vi "Run.vi"(8 "error in (no error)":errorcluster, 9 "Penalty":dbl, 10 "Maze (0: Empty, -1: Enemy. 1: Teammate":i32[][](array[numeric]), 11 "Runner in":refnum<class "Shield Wall.lvclass">) -> (0 "error out":errorcluster, 1 "Direction":T1, 2 "Action":T2, 3 "Runner out":refnum<class "Shield Wall.lvclass">, 4 "Replicated":refnum<class "Square.lvclass">)   [LabVIEW 2015, in "Shield Wall.lvclass"]
uses:
  Shield Wall.lvclass
  Type Defs/Action Enum.ctl
  Type Defs/Direction Enum.ctl
  Square/Square.lvclass
  DVR Cluster.ctl
  Shield Wall.lvclass/Shield Wall.ctl
  SubVIs/Read-Only Globals.vi
  Type Defs/SB Type Defs.lvlib
panel:
  # "NOTICE - YOU MUST NOT REMOVE THIS NOTICE. PER THE FOLLOWING LICENSE, YOU MAY REPRODUCE THIS SOFTWARE PROVIDED YOU FOLLOW THE TERMS\nOF THE LICENSE.\n\n---BEGIN BSD LICENSE (http://opensource.org/licenses/BSD-2-Clause)---\nCopyright (c) 2015, Endigit, Inc. <robert@endigit.com>\nAll rights reserved.\n\nRedistribution and use in source and binary forms, with or without modification, are permitted provided that the following conditions are met:\n\n1. Redistributions of source code must retain the above copyright notice, this list of conditions and the following disclaimer.\n\n2. Redistributions in binary form must reproduce the above copyright notice, this list of conditions and the following disclaimer in the documentation and/or other \nmaterials provided with the distribution.\n\nTHIS SOFTWARE IS PROVIDED BY THE COPYRIGHT HOLDERS AND CONTRIBUTORS \"AS IS\" AND ANY EXPRESS OR IMPLIED WARRANTIES, INCLUDING, BUT NOT \nLIMITED TO, THE IMPLIED WARRANTIES OF MERCHANTABILITY AND FITNESS FOR A PARTICULAR PURPOSE ARE DISCLAIMED. IN NO EVENT SHALL THE COPYRIGHT \nHOLDER OR CONTRIBUTORS BE LIABLE FOR ANY DIRECT, INDIRECT, INCIDENTAL, SPECIAL, EXEMPLARY, OR CONSEQUENTIAL DAMAGES (INCLUDING, BUT NOT \nLIMITED TO, PROCUREMENT OF SUBSTITUTE GOODS OR SERVICES; LOSS OF USE, DATA, OR PROFITS; OR BUSINESS INTERRUPTION) HOWEVER CAUSED AND ON \nANY THEORY OF LIABILITY, WHETHER IN CONTRACT, STRICT LIABILITY, OR TORT (INCLUDING NEGLIGENCE OR OTHERWISE) ARISING IN ANY WAY OUT OF THE USE \nOF THIS SOFTWARE, EVEN IF ADVISED OF THE POSSIBILITY OF SUCH DAMAGE.\n---END BSD LICENSE---"
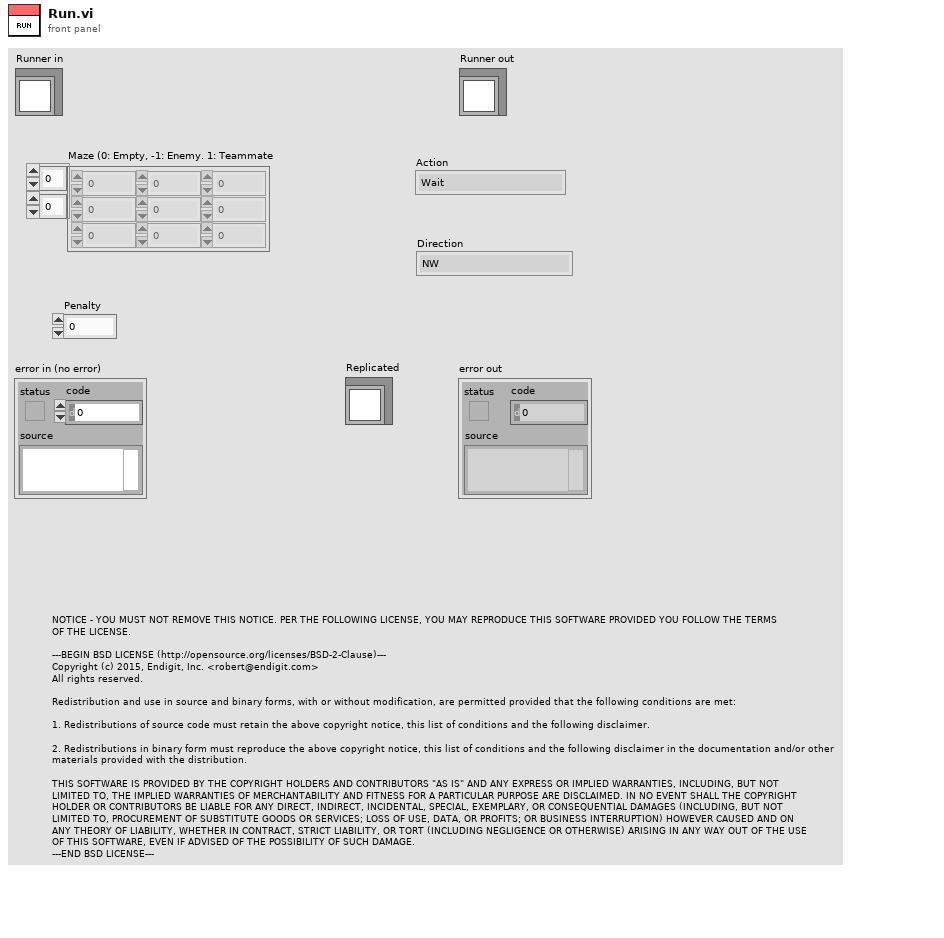
[diagram p1: front panel]
types:
  T1 = typedef "SB Type Defs.lvlib/Direction Enum.ctl" = enum16{"NW", "N", "NE", "E", "SE", "S", "SW", "W"}
  T2 = typedef "SB Type Defs.lvlib/Action Enum.ctl" = enum16{"Wait", "Move", "Attack", "Replicate"}
  T3 = typedef "Shield Wall.lvclass/DVR Cluster.ctl" = cluster{"N":i32, "E":i32, "S":i32, "W":i32, "Init":bool, "R":i32}
  T4 = typedef "Shield Wall.lvclass/Post Enum.ctl" = enum16{"NW", "NNW", "NNE", "NE", "ENE", "ESE", "SE", "SSE", "SSW", "SW", "WSW", "WNW"}
  T5 = typedef "Shield Wall.lvclass/Ring Enum.ctl" = enum16{"Defense", "Fill", "Hold", "Spawn", "Replicate", "Inner"}
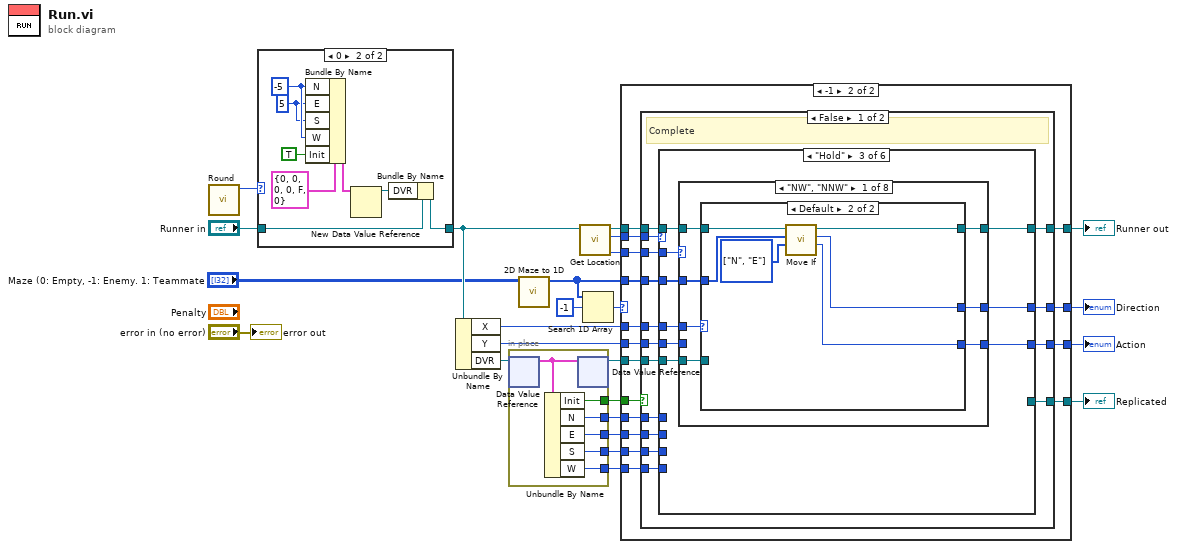
[diagram p0: block diagram]
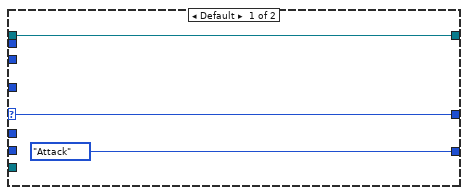
[diagram p2: hidden frame]
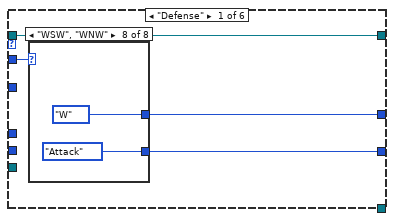
[diagram p3: hidden frame]
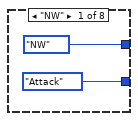
[diagram p4: hidden frame]
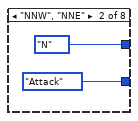
[diagram p5: hidden frame]
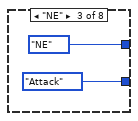
[diagram p6: hidden frame]
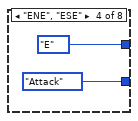
[diagram p7: hidden frame]
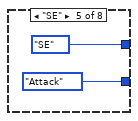
[diagram p8: hidden frame]
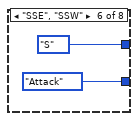
[diagram p9: hidden frame]
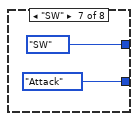
[diagram p10: hidden frame]
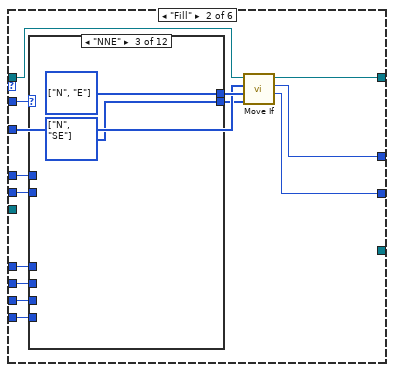
[diagram p11: hidden frame]
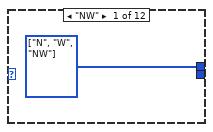
[diagram p12: hidden frame]
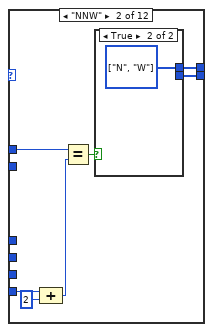
[diagram p13: hidden frame]
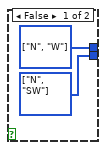
[diagram p14: hidden frame]
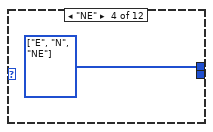
[diagram p15: hidden frame]
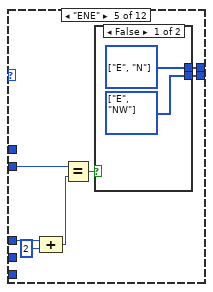
[diagram p16: hidden frame]
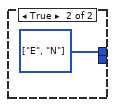
[diagram p17: hidden frame]
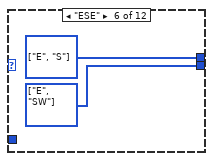
[diagram p18: hidden frame]
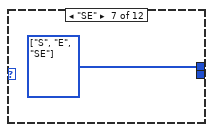
[diagram p19: hidden frame]
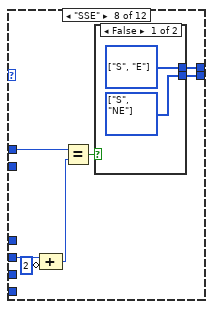
[diagram p20: hidden frame]
diagram:
  n1 = call "Round.vi"() -> ("Round"=w23:i32)  [unwired: 11 in]
  n2 = case shown="0" w23 {
    tunnel: "Runner in" -> [w25 w33]
    tunnel: [w25 w31] -> w20
    frame Default {
    }
    frame 0 {
      w27 = 5 ("E")
      w28 = -5 ("N")
      n3 = Bundle By Name(cluster=T3 {"N"=0, "E"=0, "S"=0, "W"=0, "Init"=FALSE, "R"=0} ("DVR Cluster"), "N"=w28, "E"=w27, "S"=w27, "W"=w28, "Init"=TRUE) -> (w29:T3)
      n4 = New Data Value Reference(data value=w29) -> (data value reference=w32:refnum<data-value>)  [unwired: 1 in, 1 out]
      n5 = Bundle By Name(cluster=w33, "DVR"=w32) -> (w31:refnum<class "Shield Wall.lvclass">)
    }
  }
  n6 = Unbundle By Name(w20) -> ("X"=w18:i32, "Y"=w17:i32, "DVR"=w21:refnum<data-value>)
  n7 = in-place {
    in-place-border: [w38] -> w16
    in-place-border: [w37] -> w7
    in-place-border: [w36] -> w6
    in-place-border: [w35] -> w5
    in-place-border: [w34] -> w4
    n8 = in-place-dvr #1(w21) -> (w39:T3)  [unwired: 1 out]
    n9 = Unbundle By Name(w39) -> ("Init"=w38:bool, "N"=w37:i32, "E"=w36:i32, "S"=w35:i32, "W"=w34:i32)
    n10 = in-place-dvr #1(w39) -> (w11:refnum<data-value>)  [unwired: 1 out]
  }
  n11 = call "2D Maze to 1D.vi"("Maze (0: Empty, -1: Enemy. >0: Teammate"="Maze (0: Empty, -1: Enemy. 1: Teammate") -> ("1D Maze"=w9:i32[])  [unwired: 10 in]
  n12 = call "Get Location.vi"("Class"=w20) -> ("Post"=w1:T4, "Ring"=w2:T5, "Class"=w3:refnum<class "Shield Wall.lvclass">)  [unwired: 8 in]
  n13 = Search 1D Array(1D array=w9, element=-1) -> (index of element=w8:i32)  [unwired: 1 in]
  n14 = case shown="-1" w8 {
    selector: w8 -> [w40 _]
    tunnel: w3 -> [w42 w58]
    tunnel: [w42 w57] -> w19
    tunnel: w18 -> [_ w56]
    tunnel: w17 -> [_ w55]
    tunnel: w16 -> [_ w54]
    tunnel: [w40 w53] -> w15
    tunnel: [Action_Enum."Attack" ("Action") w52] -> w14
    tunnel: [_ w51] -> w13
    tunnel: w11 -> [_ w50]
    tunnel: w9 -> [_ w49]
    tunnel: w7 -> [_ w48]
    tunnel: w6 -> [_ w47]
    tunnel: w5 -> [_ w46]
    tunnel: w4 -> [_ w45]
    tunnel: w2 -> [_ w44]
    tunnel: w1 -> [_ w43]
    frame Default {
    }
    frame -1 {
      n15 = case shown="False" w54 {
        tunnel: w58 -> [w72 w448]
        tunnel: [w73 w444] -> w57
        tunnel: w56 -> [w60 w450]
        tunnel: w55 -> [w59 w451]
        tunnel: w49 -> [w69 w449]
        tunnel: [w68 w445] -> w53
        tunnel: [w67 w446] -> w52
        tunnel: w50 -> [w65 w447]
        tunnel: [w66 w443] -> w51
        tunnel: w48 -> [w64 _]
        tunnel: w47 -> [w63 _]
        tunnel: w46 -> [w62 _]
        tunnel: w45 -> [w61 _]
        tunnel: w44 -> [w71 _]
        tunnel: w43 -> [w70 _]
        frame False {
          # "Complete"
          n16 = case shown="\"Hold\"" w71 {
            tunnel: [w77 w100 w163 w324 w343 w418] -> w73
            tunnel: w72 -> [w77 w96 w166 w320 w346 w416]
            tunnel: w70 -> [w74 w107 w168 w319 w341 _]
            tunnel: w69 -> [_ w95 w167 w321 w347 w421]
            tunnel: [w75 w99 w164 w322 w344 w420] -> w68
            tunnel: [w76 w98 w165 w323 w345 w419] -> w67
            tunnel: [_ _ _ _ w342 _] -> w66
            tunnel: w65 -> [_ _ w160 _ _ _]
            tunnel: w64 -> [_ w103 _ _ _ _]
            tunnel: w63 -> [_ w102 _ _ _ _]
            tunnel: w62 -> [_ w101 _ _ _ _]
            tunnel: w61 -> [_ w104 _ _ _ _]
            tunnel: w60 -> [_ w106 w162 _ _ _]
            tunnel: w59 -> [_ w105 w161 _ _ _]
            frame "Defense" {
              n17 = case shown="\"WSW\", \"WNW\"" w74 {
                tunnel: [Action_Enum."Attack" ("Action") Action_Enum."Attack" ("Action") Action_Enum."Attack" ("Action") Action_Enum."Attack" ("Action") Action_Enum."Attack" ("Action") Action_Enum."Attack" ("Action") Action_Enum."Attack" ("Action") Action_Enum."Attack" ("Action")] -> w76
                tunnel: [Direction_Enum."NW" ("Direction") Direction_Enum."N" ("Direction") Direction_Enum."NE" ("Direction") Direction_Enum."E" ("Direction") Direction_Enum."SE" ("Direction") Direction_Enum."S" ("Direction") Direction_Enum."SW" ("Direction") Direction_Enum."W" ("Direction")] -> w75
                frame "NW" {
                }
                frame "NNW", "NNE" {
                }
                frame "NE" {
                }
                frame "ENE", "ESE" {
                }
                frame "SE" {
                }
                frame "SSE", "SSW" {
                }
                frame "SW" {
                }
                frame "WSW", "WNW" {
                }
              }
            }
            frame "Fill" {
              n18 = case shown="\"NNE\"" w107 {
                tunnel: w106 -> [_ w113 _ _ _ _ _ w140 _ _ _ _]
                tunnel: w105 -> [_ _ _ _ w124 _ _ _ _ _ w151 _]
                tunnel: w104 -> [_ w115 _ _ _ _ _ _ _ _ _ _]
                tunnel: w103 -> [_ _ _ _ w125 _ _ _ _ _ _ _]
                tunnel: w102 -> [_ _ _ _ _ _ _ w137 _ _ _ _]
                tunnel: w101 -> [_ _ _ _ _ _ _ _ _ _ w150 _]
                tunnel: [w108 w110 w120 w121 w123 w133 w134 w136 w146 w147 w149 w159] -> w97
                tunnel: [_ w109 w119 _ w122 w132 _ w135 w145 _ w148 w158] -> w94
                frame "NW" {
                  w108 = T1[] [enum."N", enum."W", enum."NW"] items=["NW", "N", "NE", "E", "SE", "S", "SW", "W"]
                }
                frame "NNW" {
                  n19 = Compound Arithmetic op=ADD(w115, 2 ("value")) -> (w111:i32)
                  n20 = Equal?(x=w113, y=w111) -> (x = y?=w112:bool)
                  n21 = case shown="True" w112 {
                    tunnel: [w117 w118] -> w110
                    tunnel: [w116 _] -> w109
                    frame False {
                      w116 = T1[] [enum."N", enum."SW"] items=["NW", "N", "NE", "E", "SE", "S", "SW", "W"]
                      w117 = T1[] [enum."N", enum."W"] items=["NW", "N", "NE", "E", "SE", "S", "SW", "W"]
                    }
                    frame True {
                      w118 = T1[] [enum."N", enum."W"] items=["NW", "N", "NE", "E", "SE", "S", "SW", "W"]
                    }
                  }
                }
                frame "NNE" {
                  w119 = T1[] [enum."N", enum."SE"] items=["NW", "N", "NE", "E", "SE", "S", "SW", "W"]
                  w120 = T1[] [enum."N", enum."E"] items=["NW", "N", "NE", "E", "SE", "S", "SW", "W"]
                }
                frame "NE" {
                  w121 = T1[] [enum."E", enum."N", enum."NE"] items=["NW", "N", "NE", "E", "SE", "S", "SW", "W"]
                }
                frame "ENE" {
                  n22 = Compound Arithmetic op=ADD(w125, 2 ("value")) -> (w126:i32)
                  n23 = Equal?(x=w124, y=w126) -> (x = y?=w127:bool)
                  n24 = case shown="False" w127 {
                    tunnel: [w130 w131] -> w123
                    tunnel: [w129 _] -> w122
                    frame False {
                      w129 = T1[] [enum."E", enum."NW"] items=["NW", "N", "NE", "E", "SE", "S", "SW", "W"]
                      w130 = T1[] [enum."E", enum."N"] items=["NW", "N", "NE", "E", "SE", "S", "SW", "W"]
                    }
                    frame True {
                      w131 = T1[] [enum."E", enum."N"] items=["NW", "N", "NE", "E", "SE", "S", "SW", "W"]
                    }
                  }
                }
                frame "ESE" {
                  w132 = T1[] [enum."E", enum."SW"] items=["NW", "N", "NE", "E", "SE", "S", "SW", "W"]
                  w133 = T1[] [enum."E", enum."S"] items=["NW", "N", "NE", "E", "SE", "S", "SW", "W"]
                }
                frame "SE" {
                  w134 = T1[] [enum."S", enum."E", enum."SE"] items=["NW", "N", "NE", "E", "SE", "S", "SW", "W"]
                }
                frame "SSE" {
                  n25 = Compound Arithmetic op=ADD(w137, invert 2 ("value")) -> (w138:i32)
                  n26 = Equal?(x=w140, y=w138) -> (x = y?=w139:bool)
                  n27 = case shown="False" w139 {
                    tunnel: [w143 w144] -> w136
                    tunnel: [w142 _] -> w135
                    frame False {
                      w142 = T1[] [enum."S", enum."NE"] items=["NW", "N", "NE", "E", "SE", "S", "SW", "W"]
                      w143 = T1[] [enum."S", enum."E"] items=["NW", "N", "NE", "E", "SE", "S", "SW", "W"]
                    }
                    frame True {
                      w144 = T1[] [enum."S", enum."E"] items=["NW", "N", "NE", "E", "SE", "S", "SW", "W"]
                    }
                  }
                }
                frame "SSW" {
                  w145 = T1[] [enum."S", enum."NW"] items=["NW", "N", "NE", "E", "SE", "S", "SW", "W"]
                  w146 = T1[] [enum."S", enum."W"] items=["NW", "N", "NE", "E", "SE", "S", "SW", "W"]
                }
                frame "SW" {
                  w147 = T1[] [enum."W", enum."S", enum."SW"] items=["NW", "N", "NE", "E", "SE", "S", "SW", "W"]
                }
                frame "WSW" {
                  n28 = Compound Arithmetic op=ADD(w150, invert 2 ("value")) -> (w152:i32)
                  n29 = Equal?(x=w151, y=w152) -> (x = y?=w153:bool)
                  n30 = case shown="True" w153 {
                    tunnel: [w156 w157] -> w149
                    tunnel: [w155 _] -> w148
                    frame False {
                      w155 = T1[] [enum."W", enum."SE"] items=["NW", "N", "NE", "E", "SE", "S", "SW", "W"]
                      w156 = T1[] [enum."W", enum."S"] items=["NW", "N", "NE", "E", "SE", "S", "SW", "W"]
                    }
                    frame True {
                      w157 = T1[] [enum."W", enum."S"] items=["NW", "N", "NE", "E", "SE", "S", "SW", "W"]
                    }
                  }
                }
                frame "WNW" {
                  w158 = T1[] [enum."W", enum."NE"] items=["NW", "N", "NE", "E", "SE", "S", "SW", "W"]
                  w159 = T1[] [enum."W", enum."N"] items=["NW", "N", "NE", "E", "SE", "S", "SW", "W"]
                }
              }
              n31 = call "Move If.vi"("If"=w94, "Move"=w97, "1D Maze"=w95, "Shield Wall in"=w96) -> ("Action"=w98:T2, "Direction"=w99:T1, "Shield Wall out"=w100:refnum<class "Shield Wall.lvclass">)  [unwired: 5 in]
            }
            frame "Hold" {
              n32 = case shown="\"NW\", \"NNW\"" w168 {
                tunnel: w167 -> [w174 w195 w211 w233 w248 w269 w285 w307]
                tunnel: w166 -> [w175 w197 w212 w235 w249 w271 w286 w309]
                tunnel: [w173 w201 w210 w239 w247 w275 w284 w313] -> w165
                tunnel: [w172 w200 w209 w238 w246 w274 w283 w312] -> w164
                tunnel: [w171 w196 w208 w234 w245 w270 w282 w308] -> w163
                tunnel: w162 -> [w169 w202 _ _ w243 w276 _ _]
                tunnel: w161 -> [_ _ w206 w232 _ _ w280 w306]
                tunnel: w160 -> [w170 _ w207 _ w244 _ w281 _]
                frame "NW", "NNW" {
                  n33 = case shown="Default" w169 {
                    tunnel: w175 -> [w184 w194]
                    tunnel: w174 -> [w181 w190]
                    tunnel: [w176 w193] -> w173
                    tunnel: [w178 w192] -> w172
                    tunnel: [w182 w191] -> w171
                    tunnel: w170 -> [w183 _]
                    frame -1 {
                      w179 = T1[] [enum."N", enum."E"] items=["NW", "N", "NE", "E", "SE", "S", "SW", "W"]
                      w180 = T1[] [enum."N", enum."NE"] items=["NW", "N", "NE", "E", "SE", "S", "SW", "W"]
                      n34 = call "Move If.vi"("If"=w179, "Move"=w180, "1D Maze"=w181, "Shield Wall in"=w184) -> ("Action"=w177:T2, "Direction"=w178:T1, "Shield Wall out"=w182:refnum<class "Shield Wall.lvclass">)  [unwired: 5 in]
                      n35 = case shown="\"Wait\"" w177 {
                        selector: w177 -> [w185 w186]
                        tunnel: w183 -> [_ w188]
                        tunnel: [w185 w186] -> w176
                        frame Default {
                        }
                        frame "Wait" {
                          n36 = call "Push Border.vi"("Direction"=enum16{"N", "E", "S", "W"}."N", "DVR"=w188) -> ()  [unwired: 10 in]
                        }
                      }
                    }
                    frame Default {
                      w189 = T1[] [enum."N", enum."E"] items=["NW", "N", "NE", "E", "SE", "S", "SW", "W"]
                      n37 = call "Move If.vi"("Move"=w189, "1D Maze"=w190, "Shield Wall in"=w194) -> ("Action"=w193:T2, "Direction"=w192:T1, "Shield Wall out"=w191:refnum<class "Shield Wall.lvclass">)  [unwired: 6 in]
                    }
                  }
                }
                frame "NNE" {
                  n38 = case shown="0" w202 {
                    tunnel: [w204 w205] -> w199
                    tunnel: [w203 _] -> w198
                    frame 0 {
                      w203 = T1[] [enum."N", enum."W"] items=["NW", "N", "NE", "E", "SE", "S", "SW", "W"]
                      w204 = T1[] [enum."N", enum."NW"] items=["NW", "N", "NE", "E", "SE", "S", "SW", "W"]
                    }
                    frame Default {
                      w205 = T1[] [enum."N", enum."W"] items=["NW", "N", "NE", "E", "SE", "S", "SW", "W"]
                    }
                  }
                  n39 = call "Move If.vi"("If"=w198, "Move"=w199, "1D Maze"=w195, "Shield Wall in"=w197) -> ("Action"=w201:T2, "Direction"=w200:T1, "Shield Wall out"=w196:refnum<class "Shield Wall.lvclass">)  [unwired: 5 in]
                }
                frame "NE", "ENE" {
                  n40 = case shown="Default" w206 {
                    tunnel: w212 -> [w221 w231]
                    tunnel: w211 -> [w218 w227]
                    tunnel: [w213 w230] -> w210
                    tunnel: [w215 w229] -> w209
                    tunnel: [w219 w228] -> w208
                    tunnel: w207 -> [w220 _]
                    frame -1 {
                      w216 = T1[] [enum."E", enum."S"] items=["NW", "N", "NE", "E", "SE", "S", "SW", "W"]
                      w217 = T1[] [enum."E", enum."SE"] items=["NW", "N", "NE", "E", "SE", "S", "SW", "W"]
                      n41 = call "Move If.vi"("If"=w216, "Move"=w217, "1D Maze"=w218, "Shield Wall in"=w221) -> ("Action"=w214:T2, "Direction"=w215:T1, "Shield Wall out"=w219:refnum<class "Shield Wall.lvclass">)  [unwired: 5 in]
                      n42 = case shown="\"Wait\"" w214 {
                        selector: w214 -> [w222 w223]
                        tunnel: w220 -> [_ w225]
                        tunnel: [w222 w223] -> w213
                        frame Default {
                        }
                        frame "Wait" {
                          n43 = call "Push Border.vi"("Direction"=enum16{"N", "E", "S", "W"}."E", "DVR"=w225) -> ()  [unwired: 10 in]
                        }
                      }
                    }
                    frame Default {
                      w226 = T1[] [enum."E", enum."S"] items=["NW", "N", "NE", "E", "SE", "S", "SW", "W"]
                      n44 = call "Move If.vi"("Move"=w226, "1D Maze"=w227, "Shield Wall in"=w231) -> ("Action"=w230:T2, "Direction"=w229:T1, "Shield Wall out"=w228:refnum<class "Shield Wall.lvclass">)  [unwired: 6 in]
                    }
                  }
                }
                frame "ESE" {
                  n45 = case shown="0" w232 {
                    tunnel: [w241 w242] -> w237
                    tunnel: [w240 _] -> w236
                    frame 0 {
                      w240 = T1[] [enum."E", enum."N"] items=["NW", "N", "NE", "E", "SE", "S", "SW", "W"]
                      w241 = T1[] [enum."E", enum."NE"] items=["NW", "N", "NE", "E", "SE", "S", "SW", "W"]
                    }
                    frame Default {
                      w242 = T1[] [enum."E", enum."N"] items=["NW", "N", "NE", "E", "SE", "S", "SW", "W"]
                    }
                  }
                  n46 = call "Move If.vi"("If"=w236, "Move"=w237, "1D Maze"=w233, "Shield Wall in"=w235) -> ("Action"=w239:T2, "Direction"=w238:T1, "Shield Wall out"=w234:refnum<class "Shield Wall.lvclass">)  [unwired: 5 in]
                }
                frame "SE", "SSE" {
                  n47 = case shown="Default" w243 {
                    tunnel: w249 -> [w258 w268]
                    tunnel: w248 -> [w255 w264]
                    tunnel: [w250 w267] -> w247
                    tunnel: [w252 w266] -> w246
                    tunnel: [w256 w265] -> w245
                    tunnel: w244 -> [w257 _]
                    frame 1 {
                      w253 = T1[] [enum."S", enum."W"] items=["NW", "N", "NE", "E", "SE", "S", "SW", "W"]
                      w254 = T1[] [enum."S", enum."SW"] items=["NW", "N", "NE", "E", "SE", "S", "SW", "W"]
                      n48 = call "Move If.vi"("If"=w253, "Move"=w254, "1D Maze"=w255, "Shield Wall in"=w258) -> ("Action"=w251:T2, "Direction"=w252:T1, "Shield Wall out"=w256:refnum<class "Shield Wall.lvclass">)  [unwired: 5 in]
                      n49 = case shown="\"Wait\"" w251 {
                        selector: w251 -> [w259 w260]
                        tunnel: w257 -> [_ w262]
                        tunnel: [w259 w260] -> w250
                        frame Default {
                        }
                        frame "Wait" {
                          n50 = call "Push Border.vi"("Direction"=enum16{"N", "E", "S", "W"}."S", "DVR"=w262) -> ()  [unwired: 10 in]
                        }
                      }
                    }
                    frame Default {
                      w263 = T1[] [enum."S", enum."W"] items=["NW", "N", "NE", "E", "SE", "S", "SW", "W"]
                      n51 = call "Move If.vi"("Move"=w263, "1D Maze"=w264, "Shield Wall in"=w268) -> ("Action"=w267:T2, "Direction"=w266:T1, "Shield Wall out"=w265:refnum<class "Shield Wall.lvclass">)  [unwired: 6 in]
                    }
                  }
                }
                frame "SSW" {
                  n52 = case shown="-1" w276 {
                    tunnel: [w278 w279] -> w273
                    tunnel: [w277 _] -> w272
                    frame -1 {
                      w277 = T1[] [enum."S", enum."E"] items=["NW", "N", "NE", "E", "SE", "S", "SW", "W"]
                      w278 = T1[] [enum."S", enum."SE"] items=["NW", "N", "NE", "E", "SE", "S", "SW", "W"]
                    }
                    frame Default {
                      w279 = T1[] [enum."S", enum."E"] items=["NW", "N", "NE", "E", "SE", "S", "SW", "W"]
                    }
                  }
                  n53 = call "Move If.vi"("If"=w272, "Move"=w273, "1D Maze"=w269, "Shield Wall in"=w271) -> ("Action"=w275:T2, "Direction"=w274:T1, "Shield Wall out"=w270:refnum<class "Shield Wall.lvclass">)  [unwired: 5 in]
                }
                frame "SW", "WSW" {
                  n54 = case shown="Default" w280 {
                    tunnel: w286 -> [w295 w305]
                    tunnel: w285 -> [w292 w301]
                    tunnel: [w287 w304] -> w284
                    tunnel: [w289 w303] -> w283
                    tunnel: [w293 w302] -> w282
                    tunnel: w281 -> [w294 _]
                    frame 1 {
                      w290 = T1[] [enum."W", enum."N"] items=["NW", "N", "NE", "E", "SE", "S", "SW", "W"]
                      w291 = T1[] [enum."W", enum."NW"] items=["NW", "N", "NE", "E", "SE", "S", "SW", "W"]
                      n55 = call "Move If.vi"("If"=w290, "Move"=w291, "1D Maze"=w292, "Shield Wall in"=w295) -> ("Action"=w288:T2, "Direction"=w289:T1, "Shield Wall out"=w293:refnum<class "Shield Wall.lvclass">)  [unwired: 5 in]
                      n56 = case shown="\"Wait\"" w288 {
                        selector: w288 -> [w296 w297]
                        tunnel: w294 -> [_ w299]
                        tunnel: [w296 w297] -> w287
                        frame Default {
                        }
                        frame "Wait" {
                          n57 = call "Push Border.vi"("Direction"=enum16{"N", "E", "S", "W"}."W", "DVR"=w299) -> ()  [unwired: 10 in]
                        }
                      }
                    }
                    frame Default {
                      w300 = T1[] [enum."W", enum."N"] items=["NW", "N", "NE", "E", "SE", "S", "SW", "W"]
                      n58 = call "Move If.vi"("Move"=w300, "1D Maze"=w301, "Shield Wall in"=w305) -> ("Action"=w304:T2, "Direction"=w303:T1, "Shield Wall out"=w302:refnum<class "Shield Wall.lvclass">)  [unwired: 6 in]
                    }
                  }
                }
                frame "WNW" {
                  n59 = case shown="-1" w306 {
                    tunnel: [w315 w316] -> w311
                    tunnel: [w314 _] -> w310
                    frame -1 {
                      w314 = T1[] [enum."W", enum."S"] items=["NW", "N", "NE", "E", "SE", "S", "SW", "W"]
                      w315 = T1[] [enum."W", enum."SW"] items=["NW", "N", "NE", "E", "SE", "S", "SW", "W"]
                    }
                    frame Default {
                      w316 = T1[] [enum."W", enum."S"] items=["NW", "N", "NE", "E", "SE", "S", "SW", "W"]
                    }
                  }
                  n60 = call "Move If.vi"("If"=w310, "Move"=w311, "1D Maze"=w307, "Shield Wall in"=w309) -> ("Action"=w313:T2, "Direction"=w312:T1, "Shield Wall out"=w308:refnum<class "Shield Wall.lvclass">)  [unwired: 5 in]
                }
              }
            }
            frame "Spawn" {
              n61 = case shown="\"WNW\"" w319 {
                tunnel: [w326 w328 w330 w332 w334 w336 w338 w340] -> w318
                tunnel: [w325 w327 w329 w331 w333 w335 w337 w339] -> w317
                frame "NW", "NNW" {
                  w325 = T1[] [enum."SE", enum."NW"] items=["NW", "N", "NE", "E", "SE", "S", "SW", "W"]
                  w326 = T1[] [enum."SE", enum."N"] items=["NW", "N", "NE", "E", "SE", "S", "SW", "W"]
                }
                frame "NNE" {
                  w327 = T1[] [enum."SE", enum."NE"] items=["NW", "N", "NE", "E", "SE", "S", "SW", "W"]
                  w328 = T1[] [enum."SE", enum."N"] items=["NW", "N", "NE", "E", "SE", "S", "SW", "W"]
                }
                frame "NE", "ENE" {
                  w329 = T1[] [enum."SW", enum."NE"] items=["NW", "N", "NE", "E", "SE", "S", "SW", "W"]
                  w330 = T1[] [enum."SW", enum."E"] items=["NW", "N", "NE", "E", "SE", "S", "SW", "W"]
                }
                frame "ESE" {
                  w331 = T1[] [enum."SW", enum."SE"] items=["NW", "N", "NE", "E", "SE", "S", "SW", "W"]
                  w332 = T1[] [enum."SW", enum."E"] items=["NW", "N", "NE", "E", "SE", "S", "SW", "W"]
                }
                frame "SE", "SSE" {
                  w333 = T1[] [enum."NW", enum."SE"] items=["NW", "N", "NE", "E", "SE", "S", "SW", "W"]
                  w334 = T1[] [enum."NW", enum."S"] items=["NW", "N", "NE", "E", "SE", "S", "SW", "W"]
                }
                frame "SSW" {
                  w335 = T1[] [enum."NW", enum."SW"] items=["NW", "N", "NE", "E", "SE", "S", "SW", "W"]
                  w336 = T1[] [enum."NW", enum."S"] items=["NW", "N", "NE", "E", "SE", "S", "SW", "W"]
                }
                frame "SW", "WSW" {
                  w337 = T1[] [enum."NE", enum."SW"] items=["NW", "N", "NE", "E", "SE", "S", "SW", "W"]
                  w338 = T1[] [enum."NE", enum."W"] items=["NW", "N", "NE", "E", "SE", "S", "SW", "W"]
                }
                frame "WNW" {
                  w339 = T1[] [enum."NE", enum."NW"] items=["NW", "N", "NE", "E", "SE", "S", "SW", "W"]
                  w340 = T1[] [enum."NE", enum."W"] items=["NW", "N", "NE", "E", "SE", "S", "SW", "W"]
                }
              }
              n62 = call "Move If.vi"("If"=w317, "Move"=w318, "1D Maze"=w321, "Shield Wall in"=w320) -> ("Action"=w323:T2, "Direction"=w322:T1, "Shield Wall out"=w324:refnum<class "Shield Wall.lvclass">)  [unwired: 5 in]
            }
            frame "Replicate" {
              n63 = case shown="\"SE\"..\"SSW\"" w341 {
                tunnel: w347 -> [w356 w372 w388 w404]
                tunnel: w346 -> [w355 w371 w387 w403]
                tunnel: [w354 w370 w386 w402] -> w345
                tunnel: [w353 w369 w385 w401] -> w344
                tunnel: [w352 w368 w384 w400] -> w343
                tunnel: [w351 w367 w383 w399] -> w342
                frame "NW".."NNE" {
                  w348 = Direction_Enum."N" ("Direction")
                  n64 = Index Array(array=w356, index=w348) -> (element=w349:i32)
                  n65 = Equal To 0?(x=w349) -> (x = 0?=w350:bool)
                  n66 = case shown="True" w350 {
                    tunnel: w355 -> [w358 w361]
                    tunnel: [Action_Enum."Replicate" ("Action") Action_Enum."Wait" ("Action")] -> w354
                    tunnel: w348 -> [w357 w362]
                    tunnel: [w357 w362] -> w353
                    tunnel: [w358 w361] -> w352
                    tunnel: [w359 _] -> w351
                    frame True {
                      n67 = call "Update Position.vi"("Direction"=w357, "Class"=w358) -> ("Class"=w359:refnum<class "Shield Wall.lvclass">)  [unwired: 9 in]
                    }
                    frame False {
                    }
                  }
                }
                frame "NE".."ESE" {
                  w364 = Direction_Enum."E" ("Direction")
                  n68 = Index Array(array=w372, index=w364) -> (element=w365:i32)
                  n69 = Equal To 0?(x=w365) -> (x = 0?=w366:bool)
                  n70 = case shown="True" w366 {
                    tunnel: w371 -> [w374 w377]
                    tunnel: [Action_Enum."Replicate" ("Action") Action_Enum."Wait" ("Action")] -> w370
                    tunnel: w364 -> [w373 w378]
                    tunnel: [w373 w378] -> w369
                    tunnel: [w374 w377] -> w368
                    tunnel: [w375 _] -> w367
                    frame True {
                      n71 = call "Update Position.vi"("Direction"=w373, "Class"=w374) -> ("Class"=w375:refnum<class "Shield Wall.lvclass">)  [unwired: 9 in]
                    }
                    frame False {
                    }
                  }
                }
                frame "SE".."SSW" {
                  w380 = Direction_Enum."S" ("Direction")
                  n72 = Index Array(array=w388, index=w380) -> (element=w381:i32)
                  n73 = Equal To 0?(x=w381) -> (x = 0?=w382:bool)
                  n74 = case shown="True" w382 {
                    tunnel: w387 -> [w390 w393]
                    tunnel: [Action_Enum."Replicate" ("Action") Action_Enum."Wait" ("Action")] -> w386
                    tunnel: w380 -> [w389 w394]
                    tunnel: [w389 w394] -> w385
                    tunnel: [w390 w393] -> w384
                    tunnel: [w391 _] -> w383
                    frame True {
                      n75 = call "Update Position.vi"("Direction"=w389, "Class"=w390) -> ("Class"=w391:refnum<class "Shield Wall.lvclass">)  [unwired: 9 in]
                    }
                    frame False {
                    }
                  }
                }
                frame "SW".."WNW" {
                  w396 = Direction_Enum."W" ("Direction")
                  n76 = Index Array(array=w404, index=w396) -> (element=w397:i32)
                  n77 = Equal To 0?(x=w397) -> (x = 0?=w398:bool)
                  n78 = case shown="True" w398 {
                    tunnel: w403 -> [w406 w409]
                    tunnel: [Action_Enum."Replicate" ("Action") Action_Enum."Wait" ("Action")] -> w402
                    tunnel: w396 -> [w405 w410]
                    tunnel: [w405 w410] -> w401
                    tunnel: [w406 w409] -> w400
                    tunnel: [w407 _] -> w399
                    frame True {
                      n79 = call "Update Position.vi"("Direction"=w405, "Class"=w406) -> ("Class"=w407:refnum<class "Shield Wall.lvclass">)  [unwired: 9 in]
                    }
                    frame False {
                    }
                  }
                }
              }
            }
            frame "Inner" {
              n80 = Unbundle By Name(w416) -> ("D"=w415:T1)
              n81 = for {
                N: 8 -> [_]
                tunnel: w421 -> [w442]
                tunnel: [w440] -> w417
                shift-right: [w438] -> _
                shift-left: w415 -> [w436]
                tunnel: [w436] -> w413
                tunnel: [w434] -> w412
                i -> [w435]
                stop <- w440 stop-if-true
                n82 = Index Array(array=w442, index=w436) -> (element=w441:i32)
                n83 = Increment(x=w436) -> (x+1=w439:i32)
                n84 = Equal To 0?(x=w441) -> (x = 0?=w440:bool)
                n85 = Compound Arithmetic op=AND(w439, 7 ("value")) -> (w438:i32)
                n86 = Greater Than 0?(x=w435) -> (x > 0?=w434:bool)
              }
              n87 = case shown="True" w417 {
                tunnel: w416 -> [w422 w433]
                tunnel: [_ w425] -> w420
                tunnel: [Action_Enum."Wait" ("Action") Action_Enum."Move" ("Action")] -> w419
                tunnel: [w422 w430] -> w418
                tunnel: w413 -> [_ w425]
                tunnel: w412 -> [_ w427]
                frame False {
                }
                frame True {
                  n88 = Decrement(x=w425) -> (x-1=w424:i32)
                  n89 = call "Update Position.vi"("Direction"=w425, "Class"=w433) -> ("Class"=w431:refnum<class "Shield Wall.lvclass">)  [unwired: 9 in]
                  n90 = Select(t=w424, s=w427, f=w425) -> (s? t:f=w426:i32)
                  n91 = Compound Arithmetic op=AND(w426, 7 ("value")) -> (w428:i32)
                  n92 = Bundle By Name(cluster=w431, "D"=w428) -> (w430:refnum<class "Shield Wall.lvclass">)
                }
              }
            }
          }
        }
        frame True {
          # "Init"
          n93 = case shown="-1" w451 {
            tunnel: w450 -> [_ w460 w524 w570]
            tunnel: w449 -> [_ w459 w523 w569]
            tunnel: w448 -> [w452 w458 w522 w568]
            tunnel: w447 -> [_ w457 w521 w567]
            tunnel: [_ w456 w520 w566] -> w446
            tunnel: [_ w455 w519 w565] -> w445
            tunnel: [w452 w454 w518 w564] -> w444
            tunnel: [_ w453 w517 w563] -> w443
            frame Default {
            }
            frame 0 {
              n94 = case shown="1" w460 {
                tunnel: w459 -> [w469 w487 w505 _]
                tunnel: w458 -> [w462 w482 w498 w516]
                tunnel: w457 -> [w464 _ w500 _]
                tunnel: [w466 w484 w502 _] -> w456
                tunnel: [w465 w483 w501 _] -> w455
                tunnel: [w463 w481 w497 w516] -> w454
                tunnel: [w461 w480 w499 _] -> w453
                frame -1 {
                  n95 = Index Array(array=w469, index=Direction_Enum."S" ("Direction")) -> (element=w467:i32)
                  n96 = case shown="0" w467 {
                    tunnel: [_ Action_Enum."Replicate" ("Action") _] -> w466
                    tunnel: [_ w471 _] -> w465
                    tunnel: w464 -> [_ _ w476]
                    tunnel: [w470 w472 w475] -> w463
                    tunnel: w462 -> [w470 w472 w475]
                    tunnel: [_ w473 _] -> w461
                    frame Default {
                    }
                    frame 0 {
                      w471 = Direction_Enum."S" ("Direction")
                      n97 = call "Update Position.vi"("Direction"=w471, "Class"=w472) -> ("Class"=w473:refnum<class "Shield Wall.lvclass">)  [unwired: 9 in]
                    }
                    frame 1 {
                      n98 = in-place {
                        n99 = in-place-dvr #2(w476) -> (w479:T3)  [unwired: 1 out]
                        n100 = Bundle By Name(cluster=w479, "Init"=FALSE) -> (w478:T3)
                        n101 = in-place-dvr #2(w478) -> ()  [unwired: 2 out]
                      }
                    }
                  }
                }
                frame 0 {
                  n102 = Index Array(array=w487, index=Direction_Enum."NW" ("Direction")) -> (element=w485:i32)
                  n103 = case shown="1" w485 {
                    tunnel: [_ Action_Enum."Replicate" ("Action") Action_Enum."Move" ("Action")] -> w484
                    tunnel: [_ w489 w493] -> w483
                    tunnel: w482 -> [w488 w490 w495]
                    tunnel: [w488 w490 w494] -> w481
                    tunnel: [_ w491 _] -> w480
                    frame Default {
                    }
                    frame 0 {
                      w489 = Direction_Enum."NW" ("Direction")
                      n104 = call "Update Position.vi"("Direction"=w489, "Class"=w490) -> ("Class"=w491:refnum<class "Shield Wall.lvclass">)  [unwired: 9 in]
                    }
                    frame 1 {
                      w493 = Direction_Enum."SE" ("Direction")
                      n105 = call "Update Position.vi"("Direction"=w493, "Class"=w495) -> ("Class"=w494:refnum<class "Shield Wall.lvclass">)  [unwired: 9 in]
                    }
                  }
                }
                frame 1 {
                  n106 = Index Array(array=w505, index=Direction_Enum."N" ("Direction")) -> (element=w503:i32)
                  n107 = case shown="0" w503 {
                    tunnel: [_ Action_Enum."Replicate" ("Action") _] -> w502
                    tunnel: [_ w507 _] -> w501
                    tunnel: w500 -> [_ _ w512]
                    tunnel: [_ w509 _] -> w499
                    tunnel: w498 -> [w506 w508 w511]
                    tunnel: [w506 w508 w511] -> w497
                    frame Default {
                    }
                    frame 0 {
                      w507 = Direction_Enum."N" ("Direction")
                      n108 = call "Update Position.vi"("Direction"=w507, "Class"=w508) -> ("Class"=w509:refnum<class "Shield Wall.lvclass">)  [unwired: 9 in]
                    }
                    frame 1 {
                      n109 = in-place {
                        n110 = in-place-dvr #3(w512) -> (w515:T3)  [unwired: 1 out]
                        n111 = Bundle By Name(cluster=w515, "Init"=FALSE) -> (w514:T3)
                        n112 = in-place-dvr #3(w514) -> ()  [unwired: 2 out]
                      }
                    }
                  }
                }
                frame Default {
                }
              }
            }
            frame -1 {
              n113 = case shown="-1" w524 {
                tunnel: w523 -> [w526 _]
                tunnel: w522 -> [w529 w559]
                tunnel: w521 -> [w531 w558]
                tunnel: [w533 _] -> w520
                tunnel: [w532 _] -> w519
                tunnel: [w530 w559] -> w518
                tunnel: [w528 _] -> w517
                frame -1 {
                  n114 = Index Array(array=w526, index=Direction_Enum."E" ("Direction")) -> (element=w525:i32)
                  n115 = Index Array(array=w526, index=Direction_Enum."S" ("Direction")) -> (element=w534:i32)
                  n116 = case shown="1" w534 {
                    tunnel: [_ Action_Enum."Replicate" ("Action") w542] -> w533
                    tunnel: [_ w537 w543] -> w532
                    tunnel: w531 -> [_ _ w547]
                    tunnel: [w536 w538 w544] -> w530
                    tunnel: w529 -> [w536 w538 w545]
                    tunnel: [_ w539 w541] -> w528
                    tunnel: w525 -> [_ _ w546]
                    frame Default {
                    }
                    frame 0 {
                      w537 = Direction_Enum."S" ("Direction")
                      n117 = call "Update Position.vi"("Direction"=w537, "Class"=w538) -> ("Class"=w539:refnum<class "Shield Wall.lvclass">)  [unwired: 9 in]
                    }
                    frame 1 {
                      n118 = case shown="0" w546 {
                        tunnel: w547 -> [_ _ w554]
                        tunnel: w545 -> [w551 w552 w553]
                        tunnel: [w551 w552 w553] -> w544
                        tunnel: [w550 _ _] -> w543
                        tunnel: [Action_Enum."Replicate" ("Action") _ _] -> w542
                        tunnel: [w548 _ _] -> w541
                        frame 0 {
                          w550 = Direction_Enum."E" ("Direction")
                          n119 = call "Update Position.vi"("Direction"=w550, "Class"=w551) -> ("Class"=w548:refnum<class "Shield Wall.lvclass">)  [unwired: 9 in]
                        }
                        frame Default {
                        }
                        frame 1 {
                          n120 = in-place {
                            n121 = in-place-dvr #4(w554) -> (w557:T3)  [unwired: 1 out]
                            n122 = Bundle By Name(cluster=w557, "Init"=FALSE) -> (w556:T3)
                            n123 = in-place-dvr #4(w556) -> ()  [unwired: 2 out]
                          }
                        }
                      }
                    }
                  }
                }
                frame Default {
                  n124 = in-place {
                    n125 = in-place-dvr #5(w558) -> (w562:T3)  [unwired: 1 out]
                    n126 = Bundle By Name(cluster=w562, "Init"=FALSE) -> (w561:T3)
                    n127 = in-place-dvr #5(w561) -> ()  [unwired: 2 out]
                  }
                }
              }
            }
            frame 1 {
              n128 = case shown="1" w570 {
                tunnel: w569 -> [w572 _]
                tunnel: w568 -> [w575 w605]
                tunnel: w567 -> [w577 w604]
                tunnel: [w579 _] -> w566
                tunnel: [w578 _] -> w565
                tunnel: [w576 w605] -> w564
                tunnel: [w574 _] -> w563
                frame 1 {
                  n129 = Index Array(array=w572, index=Direction_Enum."W" ("Direction")) -> (element=w571:i32)
                  n130 = Index Array(array=w572, index=Direction_Enum."N" ("Direction")) -> (element=w580:i32)
                  n131 = case shown="1" w580 {
                    tunnel: [_ Action_Enum."Replicate" ("Action") w588] -> w579
                    tunnel: [_ w583 w589] -> w578
                    tunnel: w577 -> [_ _ w593]
                    tunnel: [w582 w584 w590] -> w576
                    tunnel: w575 -> [w582 w584 w591]
                    tunnel: [_ w585 w587] -> w574
                    tunnel: w571 -> [_ _ w592]
                    frame Default {
                    }
                    frame 0 {
                      w583 = Direction_Enum."N" ("Direction")
                      n132 = call "Update Position.vi"("Direction"=w583, "Class"=w584) -> ("Class"=w585:refnum<class "Shield Wall.lvclass">)  [unwired: 9 in]
                    }
                    frame 1 {
                      n133 = case shown="1" w592 {
                        tunnel: w593 -> [_ _ w600]
                        tunnel: w591 -> [w597 w598 w599]
                        tunnel: [w597 w598 w599] -> w590
                        tunnel: [w596 _ _] -> w589
                        tunnel: [Action_Enum."Replicate" ("Action") _ _] -> w588
                        tunnel: [w594 _ _] -> w587
                        frame 0 {
                          w596 = Direction_Enum."W" ("Direction")
                          n134 = call "Update Position.vi"("Direction"=w596, "Class"=w597) -> ("Class"=w594:refnum<class "Shield Wall.lvclass">)  [unwired: 9 in]
                        }
                        frame Default {
                        }
                        frame 1 {
                          n135 = in-place {
                            n136 = in-place-dvr #6(w600) -> (w603:T3)  [unwired: 1 out]
                            n137 = Bundle By Name(cluster=w603, "Init"=FALSE) -> (w602:T3)
                            n138 = in-place-dvr #6(w602) -> ()  [unwired: 2 out]
                          }
                        }
                      }
                    }
                  }
                }
                frame Default {
                  n139 = in-place {
                    n140 = in-place-dvr #7(w604) -> (w608:T3)  [unwired: 1 out]
                    n141 = Bundle By Name(cluster=w608, "Init"=FALSE) -> (w607:T3)
                    n142 = in-place-dvr #7(w607) -> ()  [unwired: 2 out]
                  }
                }
              }
            }
          }
        }
      }
    }
  }
  "Runner out" <- w19
  "Action" <- w14
  "Direction" <- w15
  "Replicated" <- w13
  "error out" <- "error in (no error)"
